vi "Coordinate_Average_and_Transform.vi"(11 "data":dbl[][](array[numeric])) -> (3 "Array":dbl[](array[numeric]))   [LabVIEW 2016]
uses:
  <vilib>/Analysis/baseanly.llb/Mean (DBL).vi
  <vilib>/Analysis/NI_AALBase.lvlib
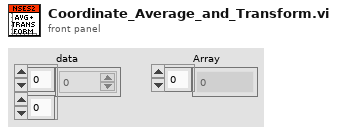
[diagram p1: front panel]
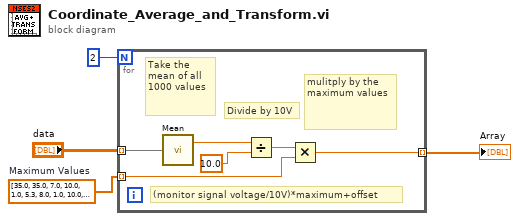
[diagram p0: block diagram]
diagram:
  w2 = dbl[] [35.0, 35.0, 7.0, 10.0, 1.0, 5.3, 8.0, 1.0, 10.0, 90.0]  # Maximum Values
  n1 = for {
    N: 2 -> [_]
    tunnel: "data" -> [w10] mode=indexing
    tunnel: [w5] -> w1 mode=indexing
    tunnel: w2 -> [w7] mode=indexing
    # "(monitor signal voltage/10V)*maximum+offset"
    # "mulitply by the maximum values"
    # "Divide by 10V"
    # "Take the mean of all 1000 values"
    n2 = call-poly <vilib>:"Mean.vi"("X"=w10) -> ("mean"=w6:dbl)  [unwired: 1 out]
    n3 = Divide(x=w6, y=10.0) -> (x/y=w8:dbl)
    n4 = Multiply(x=w8, y=w7) -> (x*y=w5:dbl)
  }
  "Array" <- w1
